vi "AddUser-Windows.vi"(8 "error in":errorcluster) -> (0 "error out":errorcluster)   [LabVIEW 2017, in "Login-UI.lvlib"]
uses:
  Login-UI.lvlib
  User-Role.ctl
  User-Info.ctl
panel:
  in  "Exit":bool
  in  "Save":bool
  in  "权  限":T1
  in  "密  码":string
  in  "用户名":string
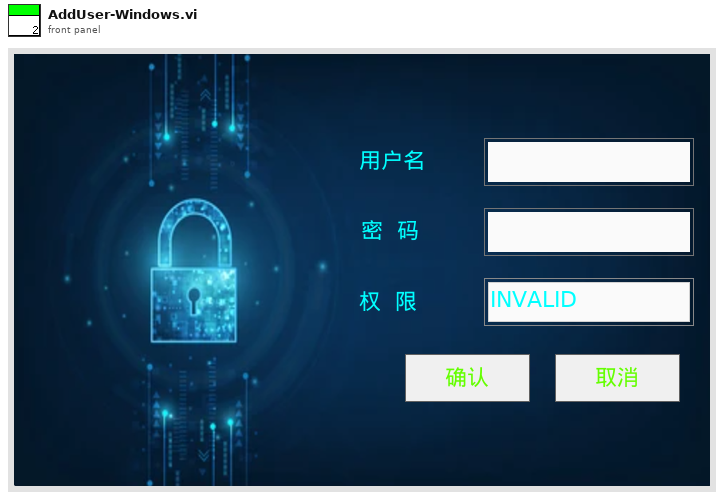
[diagram p1: front panel]
types:
  T1 = typedef "Login-UI.lvlib/User-Role.ctl" = enum16{"INVALID", "Operator", "Engineer", "Admin"}
  T2 = enum32{"Invalid", "Standard", "Closed", "Hidden", "Minimized", "Maximized"}
  T3 = enum32{"invalid app kind", "Development System", "Run Time System", "Student Edition", "Embedded LabVIEW", "Evaluation", "Custom"}
  T4 = typedef "Login-UI.lvlib/User-Info.ctl" = cluster{"UserName":string, "Password":string, "Role":T1}
  T5 = cluster{"Core":cluster{"Current VI Reference":refnum<vi>, "Close Panel on Exit?":bool}, "Your Boolean data":bool, "Your string data":string, "Cluster":T4}
  T6 = typedef "eventvkey.ctl" = enum16{"ASCII", "Enter", "Return", "Shift", "Ctrl", "Alt", "Cmd", "Opt", "Caps", "NumLock", "Clear", "Break", "Up", "Down", "Left", "Right", "Insert", "Delete", "Home", "End", "PageUp", "PageDown", "Escape", "Help", "Pause", "ScrollLock", "F1", "F2", "F3", "F4", "F5", "F6", "F7", "F8", "F9", "F10", "F11", "F12", "F13", "F14", "F15", "F16", "F17", "F18", "F19", "F20", "F21", "F22", "F23", "F24", "Play", "VolumeUp", "VolumeDown", "Mute", "Two Byte Char"}
  T7 = cluster{"Current VI Reference":refnum<vi>, "Close Panel on Exit?":bool}
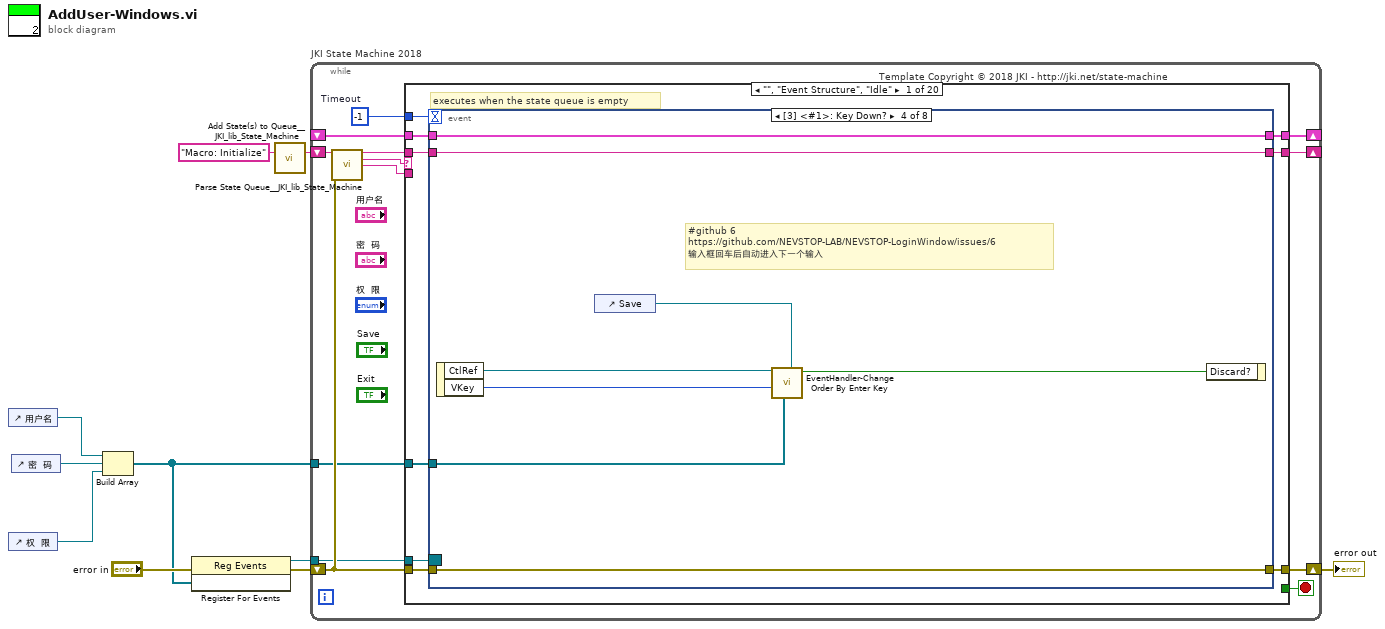
[diagram p0: block diagram]
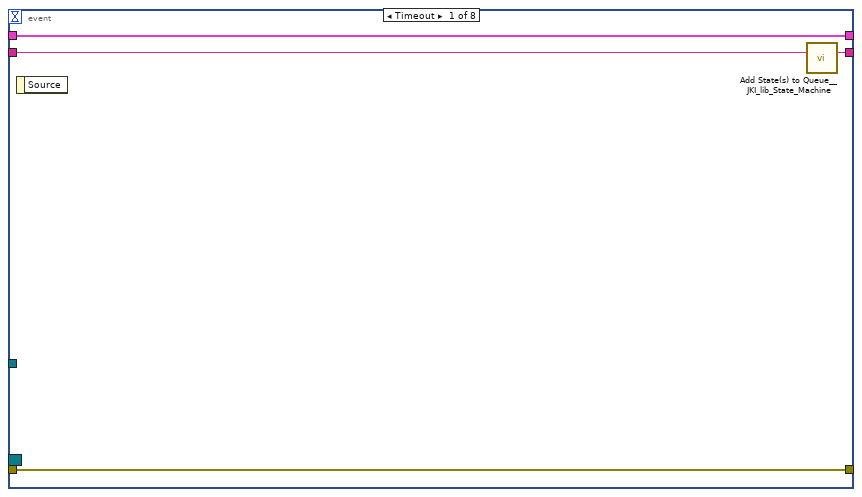
[diagram p2: hidden frame]
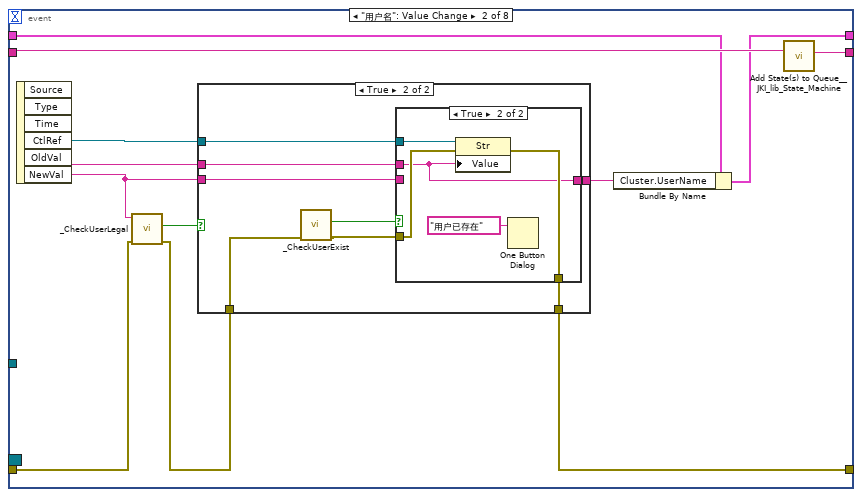
[diagram p3: hidden frame]
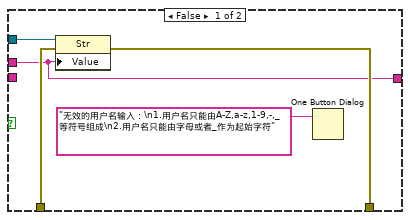
[diagram p4: hidden frame]
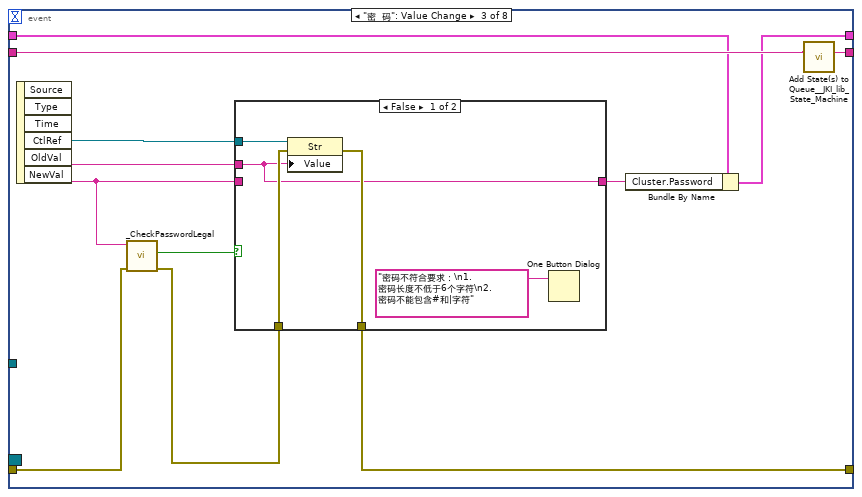
[diagram p6: hidden frame]
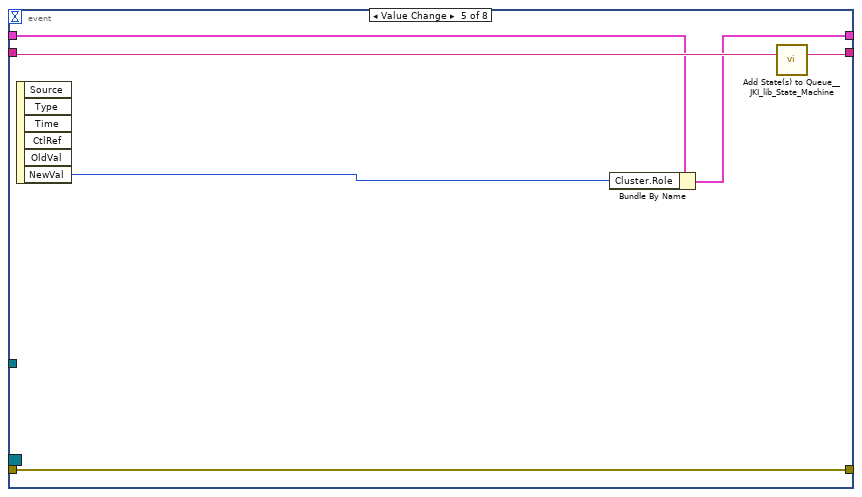
[diagram p8: hidden frame]
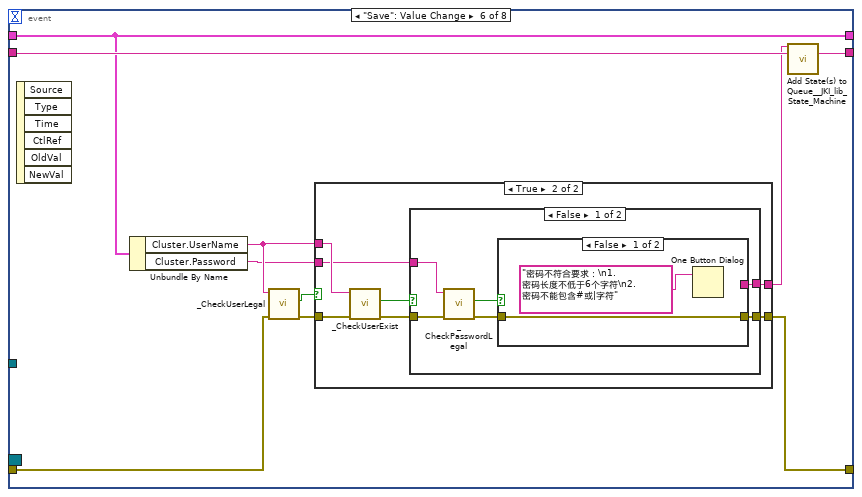
[diagram p9: hidden frame]
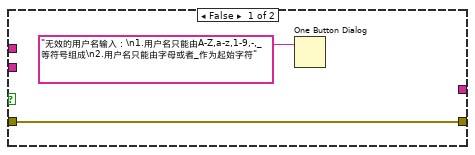
[diagram p10: hidden frame]
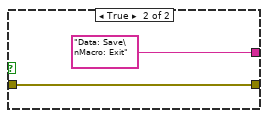
[diagram p11: hidden frame]
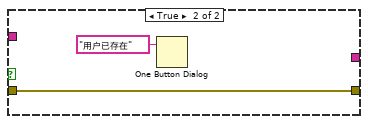
[diagram p12: hidden frame]
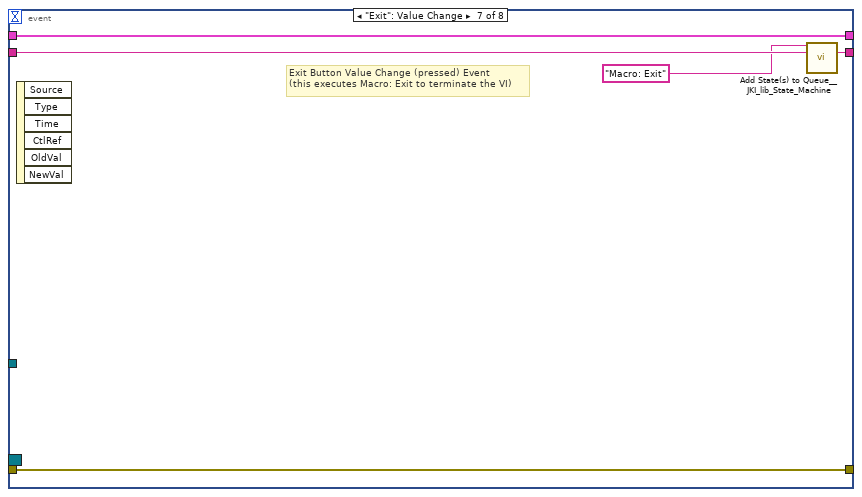
[diagram p13: hidden frame]
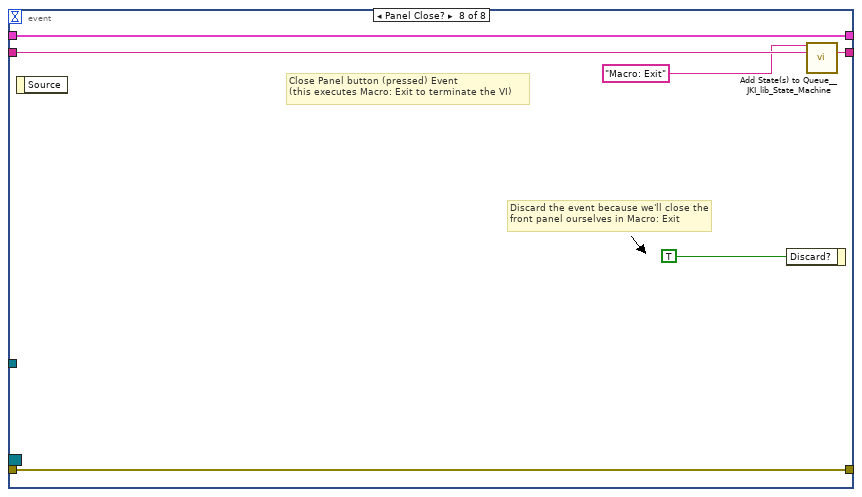
[diagram p14: hidden frame]
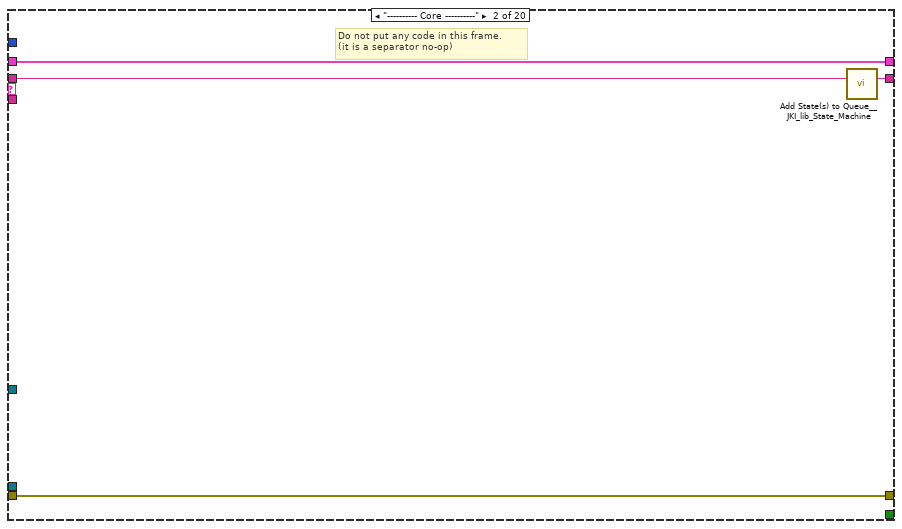
[diagram p15: hidden frame]
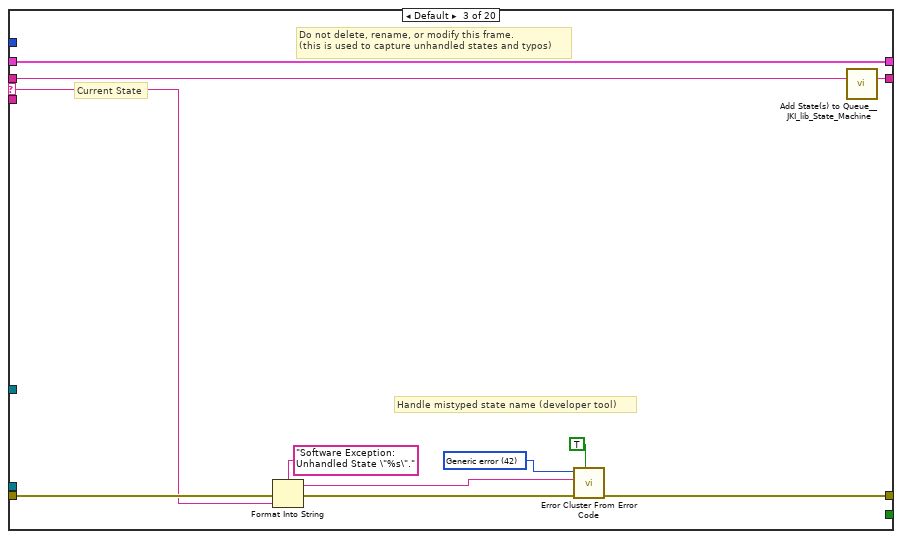
[diagram p16: hidden frame]
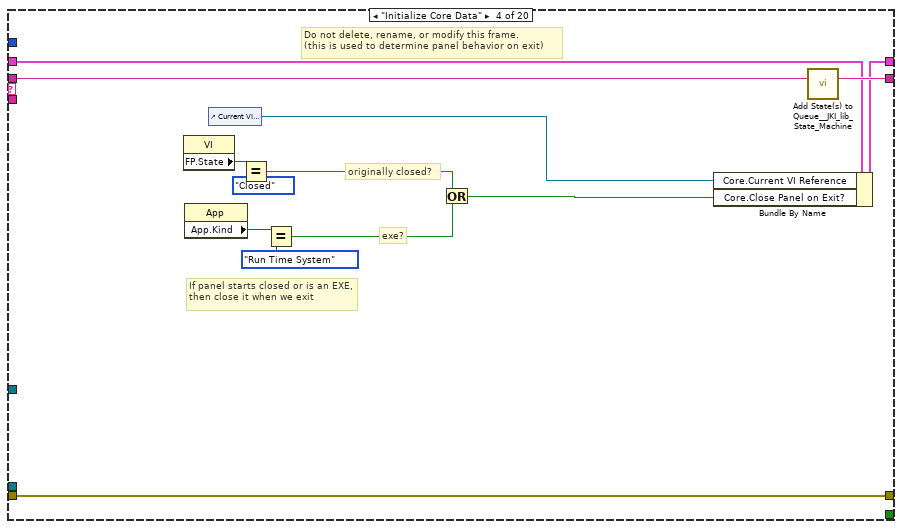
[diagram p17: hidden frame]
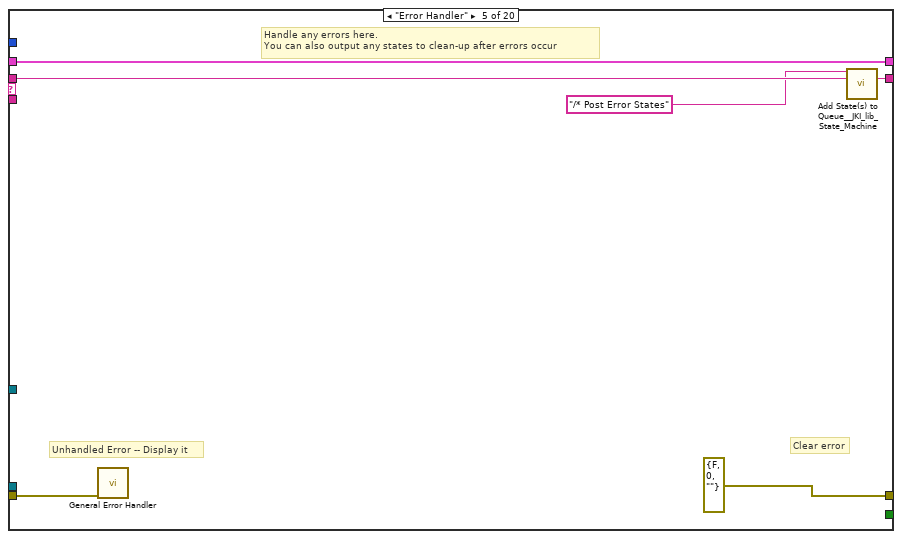
[diagram p18: hidden frame]
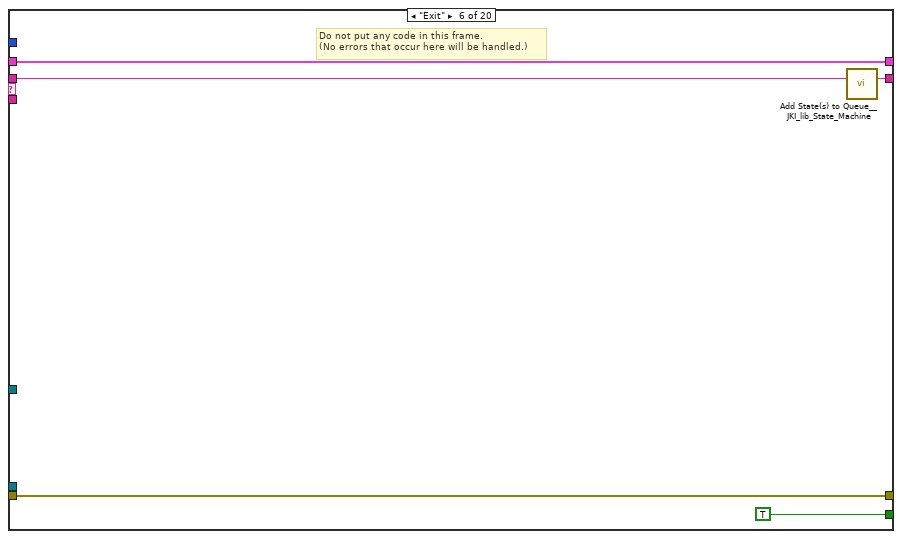
[diagram p19: hidden frame]
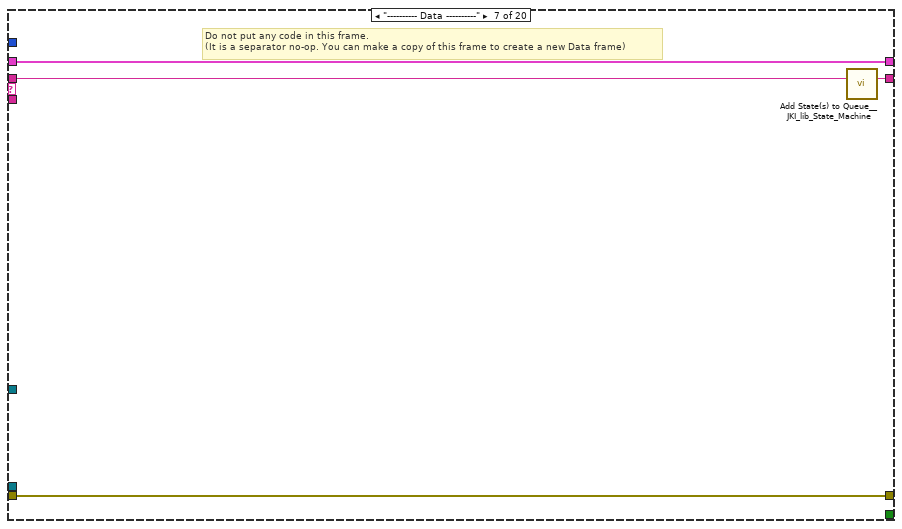
[diagram p20: hidden frame]
diagram:
  n1 = control-ref of="用户名"() -> (w1:refnum<vi>)
  n2 = control-ref of="权  限"() -> (w6:refnum<vi>)
  n3 = control-ref of="密  码"() -> (w2:refnum<vi>)
  n4 = Build Array(w1, w2, w6) -> (w3:refnum<vi>[])
  n5 = register-events(error in="error in", w3) -> (reference out=w4:refnum<event-registration>, error out=w5:errorcluster)  [unwired: 1 in]
  n6 = call <vilib>:"Add State(s) to Queue__JKI_lib_State_Machine.vi"("State(s) in (\"\")"="Macro: Initialize") -> ("States Out"=w10:string)  [unwired: 14 in]
  n7 = while "JKI State Machine 2018" {
    shift-right: [w16] -> _
    shift-left: _ -> [w15]
    shift-right: [w19] -> w7
    shift-left: w5 -> [w13]
    shift-right: [w18] -> _
    shift-left: w10 -> [w20]
    tunnel: w4 -> [w12]
    tunnel: w3 -> [w11]
    stop <- w17 stop-if-true
    w14 = -1  # Timeout
    # "Template Copyright © 2018 JKI - http://jki.net/state-machine"
    n8 = call <vilib>:"Parse State Queue__JKI_lib_State_Machine.vi"("State Queue"=w20, "Error In (no error)"=w13) -> ("Remaining States"=w22:string, "Current State"=w23:string, "Arguments"=w21:string)  [unwired: 11 in]
    n9 = case shown="\"\", \"Event Structure\", \"Idle\"" w23 {
      selector: w23 -> [_ _ w148 _ _ _ _ _ _ _ _ _ _ _ _ _ _ _ _ _]
      tunnel: w22 -> [w32 w147 w152 w171 w177 w182 w186 w194 w202 w209 w213 w221 w227 w238 w307 w312 w322 w326 w330 w334]
      tunnel: w21 -> [_ _ _ _ _ _ _ _ _ _ _ _ w222 w232 _ _ _ _ _ _]
      tunnel: w15 -> [w31 w144 w150 w164 w174 w180 w183 _ w200 w204 w210 w219 w225 w234 w304 w309 w319 w323 w327 w331]
      tunnel: [w30 w145 w154 w168 errorcluster {"status"=FALSE, "code"=0, "source"=""} ("error out") w179 w184 w191 w195 w205 w211 w216 w223 w235 w305 w310 w320 w324 w328 w332] -> w19
      tunnel: w13 -> [w29 w145 w153 w168 w173 w179 w184 w191 w197 w206 w211 w217 w224 w236 w305 w310 w320 w324 w328 w332]
      tunnel: [w26 w146 w151 w170 w176 w181 w185 w193 w203 w208 w212 w220 w226 w237 w306 w311 w321 w325 w329 w333] -> w18
      tunnel: [_ _ _ _ _ TRUE _ _ _ _ _ _ _ _ _ _ _ _ _ _] -> w17
      tunnel: [w28 w144 w150 w169 w174 w180 w183 w192 w200 w204 w210 w219 w225 w234 w304 w309 w319 w323 w327 w331] -> w16
      tunnel: w14 -> [w27 _ _ _ _ _ _ _ _ _ _ _ _ _ _ _ _ _ _ _]
      tunnel: w12 -> [w25 _ _ _ _ _ _ _ _ _ _ _ _ _ _ _ _ _ _ _]
      tunnel: w11 -> [w24 _ _ _ _ _ _ _ _ _ _ _ _ _ _ _ _ _ _ _]
      frame "", "Event Structure", "Idle" {
        # "executes when the state queue is empty"
        n10 = event shown="[3] <#1>: Key Down?" {
          selector: w25 -> [_ _ _ _ _ _ _ _]
          dyn-events: _ -> [_ _ _ _ _ _ _ _]
          timeout: w27 -> [_ _ _ _ _ _ _ _]
          tunnel: w32 -> [w36 w44 w76 w89 w99 w110 w137 w143]
          tunnel: [w35 w45 w77 w89 w100 w111 w136 w142] -> w26
          tunnel: w31 -> [w33 w39 w71 w90 w97 w106 w134 w140]
          tunnel: [w34 w46 w78 w88 w101 w102 w135 w141] -> w30
          tunnel: w29 -> [w34 w41 w74 w88 w101 w103 w135 w141]
          tunnel: [w33 w37 w69 w90 w96 w106 w134 w140] -> w28
          tunnel: w24 -> [_ _ _ w92 _ _ _ _]
          event Timeout {
            n11 = event-data() -> ()  [unwired: 1 in, 1 out]
            n12 = call <vilib>:"Add State(s) to Queue__JKI_lib_State_Machine.vi"("State(s) in (\"\")"=w36) -> ("States Out"=w35:string)  [unwired: 14 in]
          }
          event "用户名": Value Change {
            n13 = event-data() -> ("CtlRef"=w48:refnum<vi>, "OldVal"=w47:string, "NewVal"=w42:string)  [unwired: 1 in, 3 out]
            n14 = call "_CheckUserLegal.vi"("error in (no error)"=w41, "Username"=w42) -> ("error out"=w40:errorcluster, "Legal?"=w43:bool)  [unwired: 8 in]
            n15 = case shown="True" w43 {
              tunnel: w48 -> [w52 w61]
              tunnel: w47 -> [w49 w60]
              tunnel: w42 -> [_ w55]
              tunnel: w40 -> [w51 w57]
              tunnel: [w50 w59] -> w46
              tunnel: [w49 w54] -> w38
              frame False {
                n16 = property class="Str"(reference=w52, error in=w51, "Value"=w49) -> (error out=w50:errorcluster)  [unwired: 1 out]
                n17 = One Button Dialog(message="无效的用户名输入：\n1.用户名只能由A-Z,a-z,1-9,-,_等符号组成\n2.用户名只能由字母或者_作为起始字符") -> ()  [unwired: 1 in, 1 out]
              }
              frame True {
                n18 = call "_CheckUserExist.vi"("Error in"=w57) -> ("Error out"=w56:errorcluster, "exist？"=w58:bool)  [unwired: 8 in, 1 out]
                n19 = case shown="True" w58 {
                  tunnel: w61 -> [_ w67]
                  tunnel: w60 -> [_ w64]
                  tunnel: w56 -> [w63 w66]
                  tunnel: [w63 w65] -> w59
                  tunnel: [w62 w64] -> w54
                  tunnel: w55 -> [w62 _]
                  frame False {
                  }
                  frame True {
                    n20 = property class="Str"(reference=w67, error in=w66, "Value"=w64) -> (error out=w65:errorcluster)  [unwired: 1 out]
                    n21 = One Button Dialog(message="用户已存在") -> ()  [unwired: 1 in, 1 out]
                  }
                }
              }
            }
            n22 = Bundle By Name(cluster=w39, "Cluster.UserName"=w38) -> (w37:T5)
            n23 = call <vilib>:"Add State(s) to Queue__JKI_lib_State_Machine.vi"("State(s) in (\"\")"=w44) -> ("States Out"=w45:string)  [unwired: 14 in]
          }
          event "密  码": Value Change {
            n24 = event-data() -> ("CtlRef"=w79:refnum<vi>, "OldVal"=w80:string, "NewVal"=w75:string)  [unwired: 1 in, 3 out]
            n25 = call "_CheckPasswordLegal.vi"("error in (no error)"=w74, "Password"=w75) -> ("error out"=w73:errorcluster, "legal?"=w72:bool)  [unwired: 8 in]
            n26 = case shown="False" w72 {
              tunnel: w80 -> [w81 _]
              tunnel: w75 -> [_ w86]
              tunnel: [w84 w87] -> w78
              tunnel: w79 -> [w83 _]
              tunnel: w73 -> [w82 w87]
              tunnel: [w81 w86] -> w70
              frame False {
                n27 = property class="Str"(reference=w83, error in=w82, "Value"=w81) -> (error out=w84:errorcluster)  [unwired: 1 out]
                n28 = One Button Dialog(message="密码不符合要求：\n1.密码长度不低于6个字符\n2. 密码不能包含#和|字符") -> ()  [unwired: 1 in, 1 out]
              }
              frame True {
              }
            }
            n29 = Bundle By Name(cluster=w71, "Cluster.Password"=w70) -> (w69:T5)
            n30 = call <vilib>:"Add State(s) to Queue__JKI_lib_State_Machine.vi"("State(s) in (\"\")"=w76) -> ("States Out"=w77:string)  [unwired: 14 in]
          }
          event Key Down? {
            # "#github 6\nhttps://github.com/NEVSTOP-LAB/NEVSTOP-LoginWindow/issues/6\n输入框回车后自动进入下一个输入"
            n31 = event-data() -> ("CtlRef"=w95:refnum<vi>, "VKey"=w94:T6)  [unwired: 1 in]
            n32 = control-ref of="Save"() -> (w93:refnum<vi>)
            n33 = call "EventHandler-Change Order By Enter Key.vi"("Next Ctrl"=w93, "Controls for changing order"=w92, "VKey"=w94, "Event Control"=w95) -> ("Discard?"=w91:bool)  [unwired: 7 in]
            n34 = event-data("Discard?"=w91) -> ()  [unwired: 1 in, 1 out]
          }
          event Value Change {
            n35 = event-data() -> ("NewVal"=w98:T1)  [unwired: 1 in, 5 out]
            n36 = Bundle By Name(cluster=w97, "Cluster.Role"=w98) -> (w96:T5)
            n37 = call <vilib>:"Add State(s) to Queue__JKI_lib_State_Machine.vi"("State(s) in (\"\")"=w99) -> ("States Out"=w100:string)  [unwired: 14 in]
          }
          event "Save": Value Change {
            n38 = event-data() -> ()  [unwired: 1 in, 6 out]
            n39 = Unbundle By Name(w106) -> ("Cluster.UserName"=w108:string, "Cluster.Password"=w107:string)
            n40 = call "_CheckUserLegal.vi"("error in (no error)"=w103, "Username"=w108) -> ("error out"=w104:errorcluster, "Legal?"=w109:bool)  [unwired: 8 in]
            n41 = case shown="True" w109 {
              tunnel: w108 -> [_ w120]
              tunnel: w107 -> [_ w118]
              tunnel: [_ w117] -> w105
              tunnel: w104 -> [w113 w116]
              tunnel: [w113 w114] -> w102
              frame False {
                n42 = One Button Dialog(message="无效的用户名输入：\n1.用户名只能由A-Z,a-z,1-9,-,_等符号组成\n2.用户名只能由字母或者_作为起始字符") -> ()  [unwired: 1 in, 1 out]
              }
              frame True {
                n43 = call "_CheckUserExist.vi"("Error in"=w116, "Username"=w120) -> ("Error out"=w115:errorcluster, "exist？"=w119:bool)  [unwired: 7 in, 1 out]
                n44 = case shown="False" w119 {
                  tunnel: w118 -> [w126 _]
                  tunnel: [w125 _] -> w117
                  tunnel: w115 -> [w124 w132]
                  tunnel: [w122 w132] -> w114
                  frame False {
                    n45 = call "_CheckPasswordLegal.vi"("error in (no error)"=w124, "Password"=w126) -> ("error out"=w121:errorcluster, "legal?"=w123:bool)  [unwired: 8 in]
                    n46 = case shown="False" w123 {
                      tunnel: [_ "Data: Save\nMacro: Exit"] -> w125
                      tunnel: [w128 w129] -> w122
                      tunnel: w121 -> [w128 w129]
                      frame False {
                        n47 = One Button Dialog(message="密码不符合要求：\n1.密码长度不低于6个字符\n2. 密码不能包含#或|字符") -> ()  [unwired: 1 in, 1 out]
                      }
                      frame True {
                      }
                    }
                  }
                  frame True {
                    n48 = One Button Dialog(message="用户已存在") -> ()  [unwired: 1 in, 1 out]
                  }
                }
              }
            }
            n49 = call <vilib>:"Add State(s) to Queue__JKI_lib_State_Machine.vi"("State(s) in Front (\"\")"=w105, "State(s) in (\"\")"=w110) -> ("States Out"=w111:string)  [unwired: 13 in]
          }
          event "Exit": Value Change {
            # "Exit Button Value Change (pressed) Event\n(this executes Macro: Exit to terminate the VI)"
            n50 = event-data() -> ()  [unwired: 1 in, 6 out]
            n51 = call <vilib>:"Add State(s) to Queue__JKI_lib_State_Machine.vi"("State(s) in Front (\"\")"="Macro: Exit", "State(s) in (\"\")"=w137) -> ("States Out"=w136:string)  [unwired: 13 in]
          }
          event Panel Close? {
            # "Discard the event because we'll close the front panel ourselves in Macro: Exit"
            # "Close Panel button (pressed) Event\n(this executes Macro: Exit to terminate the VI)"
            n52 = event-data() -> ()  [unwired: 1 in, 1 out]
            n53 = event-data("Discard?"=TRUE) -> ()  [unwired: 1 in, 1 out]
            n54 = call <vilib>:"Add State(s) to Queue__JKI_lib_State_Machine.vi"("State(s) in Front (\"\")"="Macro: Exit", "State(s) in (\"\")"=w143) -> ("States Out"=w142:string)  [unwired: 13 in]
          }
        }
      }
      frame "---------- Core ----------" {
        # "Do not put any code in this frame.\n(it is a separator no-op)"
        n55 = call <vilib>:"Add State(s) to Queue__JKI_lib_State_Machine.vi"("State(s) in (\"\")"=w147) -> ("States Out"=w146:string)  [unwired: 14 in]
      }
      frame Default {
        w157 = 42 items=["No error", "Argument error", "Memory is full", "Out of zone", "End of file", "File already open", "Generic file I/O error", "File not found", "File permission error", "Disk is full", "Duplicate path", "Too many files open", "System feature not enabled", "Resource file not found", "Cannot add resource", "Resource not found", "Image not found", "Image memory error", "Pen does not exist", "Config type invalid", "Config token not found", "Config parse error", "Config memory error", "Bad external code format", "Bad external code offset", "External code not present", "Null window", "Destroy window error", "Null menu", "Print aborted", "Bad print record", "Print driver error", "Windows error during printing", "Memory error during printing", "Print dialog error", "Generic print error", "Invalid device refnum", "Device not found", "Device parameter error", "Device unit error", "Cannot open device", "Device call aborted", "Generic error", "Cancelled by user", "Object ID too low", "Object ID too high", "Object not in heap", "Unknown heap", "Unknown object (invalid DefProc)", "Unknown object (DefProc not in table)", "Message out of range", "Invalid (null) method", "Unknown message", "Manager call not supported", "Bad address", "Network operation in progress", "Network operation timed out", "Connection is busy", "Network attribute not supported", "Network error", "Address in use", "System out of memory", "Connection aborted", "Connection refused", "Not connected", "Already connected", "Connection closed", "Initialization error (interapplication manager)", "Bad occurrence", "Wait on unbound occurrence handler", "Occurrence queue overflow", "Datalog type conflict", "Unused", "Unrecognized type (interapplication manager)", "Memory corrupt", "Failed to make temporary DLL", "Old CIN version", "Drag socket not found", "Failed to load drop-object", "Failed to register OLE object", "Failed to release OLE object", "Format specifier type mismatch", "Unknown format specifier", "Too few format specifiers", "Too many format specifiers", "Scan failed", "Newer CIN version", "Error converting to variant", "Runtime menu error", "Password tampered", "Variant attribute not found", "Incompatible variant data type", "Event data is not available", "Event Store is not present", "Occurrence is not found", "Event Queue is not created", "Event info is not available", "Refnum passed is NULL", "Error retrieving Class GUID", "Error retrieving CoClass GUID", "Error retrieving TypeLib GUID.", "Bad built application magic bytes.", "Specific driver is different from the specific driver associated with the Logical Name.", "There is no session opened to the class driver.", "Max Error", "MAX - Error with config objects", "MAX - Error loading configuration", "MAX - Group not supported"]
        # "Current State"
        # "Do not delete, rename, or modify this frame.\n(this is used to capture unhandled states and typos)"
        # "Handle mistyped state name (developer tool)"
        n56 = Format Into String(format string="Software Exception: Unhandled State \"%s\"." ("message"), error in=w153, w148) -> (resulting string=w156:string, error out=w155:errorcluster)  [unwired: 1 in]
        n57 = call <vilib>:"Error Cluster From Error Code.vi"("show call chain? (False)"=TRUE, "error in (no error)"=w155, "error message (\"\")"=w156, "error code (0)"=w157) -> ("error out"=w154:errorcluster)  [unwired: 5 in]
        n58 = call <vilib>:"Add State(s) to Queue__JKI_lib_State_Machine.vi"("State(s) in (\"\")"=w152) -> ("States Out"=w151:string)  [unwired: 14 in]
      }
      frame "Initialize Core Data" {
        # "Do not delete, rename, or modify this frame.\n(this is used to determine panel behavior on exit)"
        # "originally closed?"
        # "exe?"
        # "If panel starts closed or is an EXE, then close it when we exit"
        n59 = property class="VI"() -> ("FP.State"=w161:T2)  [unwired: 2 in, 2 out]
        n60 = property class="App"() -> ("App.Kind"=w167:T3)  [unwired: 2 in, 2 out]
        n61 = control-ref of="Current VI Reference"() -> (w162:refnum<vi>)
        n62 = Equal?(x=w161, y=T2."Closed" ("Front Panel Window:State")) -> (x = y?=w159:bool)
        n63 = Equal?(x=w167, y=T3."Run Time System" ("Application:Kind")) -> (x = y?=w165:bool)
        n64 = Or(x=w159, y=w165) -> (x .or. y?=w163:bool)
        n65 = Bundle By Name(cluster=w164, "Core.Current VI Reference"=w162, "Core.Close Panel on Exit?"=w163) -> (w169:T5)
        n66 = call <vilib>:"Add State(s) to Queue__JKI_lib_State_Machine.vi"("State(s) in (\"\")"=w171) -> ("States Out"=w170:string)  [unwired: 14 in]
      }
      frame "Error Handler" {
        # "Unhandled Error -- Display it"
        # "Handle any errors here.\nYou can also output any states to clean-up after errors occur"
        # "Clear error"
        n67 = call <vilib>:"General Error Handler.vi"("error in (no error)"=w173) -> ()  [unwired: 10 in, 5 out]
        n68 = call <vilib>:"Add State(s) to Queue__JKI_lib_State_Machine.vi"("State(s) in Front (\"\")"="/* Post Error States", "State(s) in (\"\")"=w177) -> ("States Out"=w176:string)  [unwired: 13 in]
      }
      frame "Exit" {
        # "Do not put any code in this frame.\n(No errors that occur here will be handled.)"
        n69 = call <vilib>:"Add State(s) to Queue__JKI_lib_State_Machine.vi"("State(s) in (\"\")"=w182) -> ("States Out"=w181:string)  [unwired: 14 in]
      }
      frame "---------- Data ----------" {
        # "Do not put any code in this frame.\n(It is a separator no-op. You can make a copy of this frame to create a new Data frame)"
        n70 = call <vilib>:"Add State(s) to Queue__JKI_lib_State_Machine.vi"("State(s) in (\"\")"=w186) -> ("States Out"=w185:string)  [unwired: 14 in]
      }
      frame "Data: Initialize" {
        w188 = T7 {"Current VI Reference"=refnum, "Close Panel on Exit?"=FALSE}  # Core
        w190 = TRUE  # Your Boolean data
        w189 = ""  # Your string data
        # "do not delete - used by framework"
        # "Add new data here."
        # "Data names and types of shift register data are defined by this bundle."
        # "Initialize the shift-register data, here.\n(data names are defined by what you wire into the bundle function)"
        n71 = Bundle("Core"=w188, "Your Boolean data"=w190, "Your string data"=w189, "Cluster"=T4 {"UserName"="", "Password"="", "Role"=enum."INVALID"}) -> (w192:T5)  [unwired: 1 in]
        n72 = call <vilib>:"Add State(s) to Queue__JKI_lib_State_Machine.vi"("State(s) in (\"\")"=w194) -> ("States Out"=w193:string)  [unwired: 14 in]
      }
      frame "Data: Save" {
        n73 = Unbundle By Name(w200) -> ("Cluster"=w199:T4)
        n74 = call "_Read Users From File.vi"("Error in"=w197) -> ("Error out"=w196:errorcluster, "Array"=w201:T4[])  [unwired: 9 in]
        n75 = Build Array (concatenate)(w201, w199) -> (w198:T4[])
        n76 = call "_Save Users to File.vi"("Error in"=w196, "Array"=w198) -> ("Error out"=w195:errorcluster)  [unwired: 9 in]
        n77 = call <vilib>:"Add State(s) to Queue__JKI_lib_State_Machine.vi"("State(s) in (\"\")"=w202) -> ("States Out"=w203:string)  [unwired: 14 in]
      }
      frame "Data: Cleanup" {
        # "Cleanup any data and references, here.\n(this is called automatically, by the Macro: Exit)"
        n78 = Unbundle By Name(w204) -> ("Core.Current VI Reference"=w207:refnum<vi>)
        n79 = Close Reference(reference=w207, error in (no error)=w206) -> (error out=w205:errorcluster)
        n80 = call <vilib>:"Add State(s) to Queue__JKI_lib_State_Machine.vi"("State(s) in (\"\")"=w209) -> ("States Out"=w208:string)  [unwired: 14 in]
      }
      frame "---------- UI ----------" {
        # "Do not put any code in this frame.\n(It is a separator no-op. You can make a copy of this frame to create a new UI frame)"
        n81 = call <vilib>:"Add State(s) to Queue__JKI_lib_State_Machine.vi"("State(s) in (\"\")"=w213) -> ("States Out"=w212:string)  [unwired: 14 in]
      }
      frame "UI: Initialize" {
        # "Initialize the User Interface, here.\n(this is called automatically, by the Macro: Init)"
        n82 = call <userlib>:"Fit VI window to Visible Content_nevstop.vi"("error in (no error)"=w217, "border spacing (2 px)"=-5) -> ("error out"=w215:errorcluster)  [unwired: 4 in, 1 out]
        n83 = call <userlib>:"MGI Center Callee in Caller.vi"("Error In"=w215) -> ("Error Out"=w214:errorcluster)  [unwired: 10 in]
        n84 = call <userlib>:"Clear All Error_nevstop.vi"("error in (no error)"=w214) -> ()  [unwired: 10 in, 1 out]
        n85 = invoke class="VI" method="Default Vals.Reinit All"(error in=w215) -> (error out=w216:errorcluster)  [unwired: 2 in, 2 out]
        n86 = call <vilib>:"Add State(s) to Queue__JKI_lib_State_Machine.vi"("State(s) in (\"\")"=w221) -> ("States Out"=w220:string)  [unwired: 14 in]
      }
      frame "UI: Cursor Set" {
        # "Argument"
        # "Set and Unset Cursor Busy.\n(Usage: \"UI: Cursor Set >> Busy|Idle\")"
        n87 = case shown="\"Idle\", Default" w222 {
          tunnel: w224 -> [w229 w231]
          tunnel: [w228 w230] -> w223
          frame "Idle", Default {
            n88 = call <vilib>:"Unset Busy.vi"("error in (no error)"=w229) -> ("error out"=w228:errorcluster)  [unwired: 10 in]
          }
          frame "Busy" {
            n89 = call <vilib>:"Set Busy.vi"("error in (no error)"=w231) -> ("error out"=w230:errorcluster)  [unwired: 9 in, 1 out]
          }
        }
        n90 = call <vilib>:"Add State(s) to Queue__JKI_lib_State_Machine.vi"("State(s) in (\"\")"=w227) -> ("States Out"=w226:string)  [unwired: 14 in]
      }
      frame "UI: Front Panel State" {
        # "Argument"
        # "Set Front Panel Open or Closed\n(Usage: \"UI: Front Panel State >> Open|Close\")"
        n91 = Unbundle By Name(w234) -> ("Core.Current VI Reference"=w233:refnum<vi>)
        n92 = case shown="\"Minimize\", \"Minimized\"" w232 {
          tunnel: w236 -> [w244 w259 w270 w283 w296]
          tunnel: [w246 w260 w272 w285 w298] -> w235
          tunnel: w233 -> [w245 w257 w271 w284 w297]
          frame "Open", "Standard", Default {
            w239 = T2."Standard" ("State")
            n93 = property class="VI"(reference=w245, error in=w244) -> (reference out=w242:refnum<vi>, error out=w243:errorcluster, "FP.State"=w241:T2)
            n94 = Not Equal?(x=w241, y=w239) -> (x != y?=w240:bool)
            n95 = case shown="True" w240 {
              tunnel: [w250 w252] -> w246
              tunnel: w243 -> [w249 w252]
              tunnel: w242 -> [w248 _]
              tunnel: w239 -> [w247 _]
              frame True {
                n96 = invoke class="VI" method="FP.Open"(reference=w248, error in=w249, "Activate"=TRUE, "State"=w247) -> (error out=w250:errorcluster)  [unwired: 1 in, 4 out]
              }
              frame False {
              }
            }
          }
          frame "Close", "Closed" {
            n97 = property class="VI"(reference=w257, error in=w259) -> (reference out=w256:refnum<vi>, error out=w258:errorcluster, "FP.State"=w254:T2)
            n98 = Not Equal?(x=w254, y=T2."Closed" ("Front Panel Window:State")) -> (x != y?=w253:bool)
            n99 = case shown="True" w253 {
              tunnel: [w261 w264] -> w260
              tunnel: w258 -> [w261 w263]
              tunnel: w256 -> [_ w262]
              frame False {
              }
              frame True {
                n100 = invoke class="VI" method="FP.Close"(reference=w262, error in=w263) -> (error out=w264:errorcluster)  [unwired: 1 in, 2 out]
              }
            }
          }
          frame "Hidden", "Hide" {
            w265 = T2."Hidden" ("State")
            n101 = property class="VI"(reference=w271, error in=w270) -> (reference out=w268:refnum<vi>, error out=w269:errorcluster, "FP.State"=w267:T2)
            n102 = Not Equal?(x=w267, y=w265) -> (x != y?=w266:bool)
            n103 = case shown="True" w266 {
              tunnel: [w276 w277] -> w272
              tunnel: w269 -> [w275 w277]
              tunnel: w268 -> [w274 _]
              tunnel: w265 -> [w273 _]
              frame True {
                n104 = invoke class="VI" method="FP.Open"(reference=w274, error in=w275, "State"=w273) -> (error out=w276:errorcluster)  [unwired: 2 in, 4 out]
              }
              frame False {
              }
            }
          }
          frame "Minimize", "Minimized" {
            w278 = T2."Minimized" ("State")
            n105 = property class="VI"(reference=w284, error in=w283) -> (reference out=w281:refnum<vi>, error out=w282:errorcluster, "FP.State"=w280:T2)
            n106 = Not Equal?(x=w280, y=w278) -> (x != y?=w279:bool)
            n107 = case shown="True" w279 {
              tunnel: [w289 w290] -> w285
              tunnel: w282 -> [w288 w290]
              tunnel: w281 -> [w287 _]
              tunnel: w278 -> [w286 _]
              frame True {
                n108 = invoke class="VI" method="FP.Open"(reference=w287, error in=w288, "State"=w286) -> (error out=w289:errorcluster)  [unwired: 2 in, 4 out]
              }
              frame False {
              }
            }
          }
          frame "Maximize", "Maximized" {
            w291 = T2."Maximized" ("State")
            n109 = property class="VI"(reference=w297, error in=w296) -> (reference out=w294:refnum<vi>, error out=w295:errorcluster, "FP.State"=w293:T2)
            n110 = Not Equal?(x=w293, y=w291) -> (x != y?=w292:bool)
            n111 = case shown="True" w292 {
              tunnel: [w302 w303] -> w298
              tunnel: w295 -> [w301 w303]
              tunnel: w294 -> [w300 _]
              tunnel: w291 -> [w299 _]
              frame True {
                n112 = invoke class="VI" method="FP.Open"(reference=w300, error in=w301, "State"=w299) -> (error out=w302:errorcluster)  [unwired: 2 in, 4 out]
              }
              frame False {
              }
            }
          }
        }
        n113 = call <vilib>:"Add State(s) to Queue__JKI_lib_State_Machine.vi"("State(s) in (\"\")"=w238) -> ("States Out"=w237:string)  [unwired: 14 in]
      }
      frame "---------- Macro ----------" {
        # "Do not put any code in this frame.\n(It is a separator no-op. You can make a copy of this frame to create a new Macro frame)"
        n114 = call <vilib>:"Add State(s) to Queue__JKI_lib_State_Machine.vi"("State(s) in (\"\")"=w307) -> ("States Out"=w306:string)  [unwired: 14 in]
      }
      frame "Macro: Initialize" {
        w308 = "Data: Initialize\nInitialize Core Data\nUI: Initialize\nUI: Front Panel State >> Open"  # Data: Initialize Initialize Core Data UI: Initialize UI: Front Panel State >> Open
        # "Initialization Macro\n(This is called once, when the VI starts)"
        n115 = call <vilib>:"Add State(s) to Queue__JKI_lib_State_Machine.vi"("State(s) in Front (\"\")"=w308, "State(s) in (\"\")"=w312) -> ("States Out"=w311:string)  [unwired: 13 in]
      }
      frame "Macro: Exit" {
        # "Exit Macro\n(This is called once, when the VI exits)"
        n116 = Unbundle By Name(w319) -> ("Core.Close Panel on Exit?"=w318:bool)
        n117 = Select(t="UI: Front Panel State >> Close", s=w318, f="") -> (s? t:f=w315:string)
        n118 = call <vilib>:"Add State(s) to Queue__JKI_lib_State_Machine.vi"("State(s) in (\"\")"=w315, "State(s) at Back (\"\")"="Data: Cleanup\nExit") -> ("States Out"=w313:string)  [unwired: 13 in]
        n119 = call <vilib>:"Add State(s) to Queue__JKI_lib_State_Machine.vi"("State(s) in Front (\"\")"=w313, "State(s) in (\"\")"=w322) -> ("States Out"=w321:string)  [unwired: 13 in]
      }
      frame "---------- New Category ----------" {
        # "Template Separator\n(You can make a copy of, or modify, this frame)"
        n120 = call <vilib>:"Add State(s) to Queue__JKI_lib_State_Machine.vi"("State(s) in (\"\")"=w326) -> ("States Out"=w325:string)  [unwired: 14 in]
      }
      frame "New Category: 1" {
        # "Your code here.\n(You can make a copy of, or modify, this frame)"
        n121 = call <vilib>:"Add State(s) to Queue__JKI_lib_State_Machine.vi"("State(s) in (\"\")"=w330) -> ("States Out"=w329:string)  [unwired: 14 in]
      }
      frame "New Category: 2" {
        # "Your code here.\n(You can make a copy of, or modify, this frame)"
        n122 = call <vilib>:"Add State(s) to Queue__JKI_lib_State_Machine.vi"("State(s) in (\"\")"=w334) -> ("States Out"=w333:string)  [unwired: 14 in]
      }
    }
  }
  "error out" <- w7
